vi "setUpdateTimestampFIFO.vi"(10 "UpdateTimestampFIFO":refnum<class "IWriteU64FIFO.lvclass">, 11 "Timestamp in":refnum<class "Timestamp.lvclass">) -> (3 "Timestamp out":refnum<class "Timestamp.lvclass">)   [LabVIEW 2016, in "RTTimestamp.lvlib" / "Timestamp.lvclass"]
uses:
  Timestamp.lvclass
  Common_RT_FPGA/IWriteU64FIFO/IWriteU64FIFO.lvclass
  Timestamp.lvclass/Timestamp.ctl
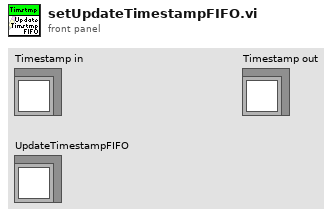
[diagram p1: front panel]
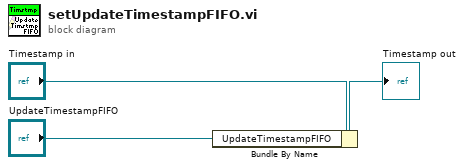
[diagram p0: block diagram]
diagram:
  n1 = Bundle By Name(cluster="Timestamp in", "UpdateTimestampFIFO"="UpdateTimestampFIFO") -> (→"Timestamp out":refnum<class "Timestamp.lvclass">)
